vi "SetTIA.vi"(8 "error in (no error)":errorcluster, 11 "Laser Diode Controller in":refnum<class "KLD101.lvclass">) -> (0 "error out":errorcluster, 3 "Laser Diode Controller out":refnum<class "KLD101.lvclass">)   [LabVIEW 2016, in "Laser Diode Controller.lvlib" / "KLD101.lvclass"]
uses:
  KLD101.lvclass
  KLD101.lvclass/KLD101.ctl
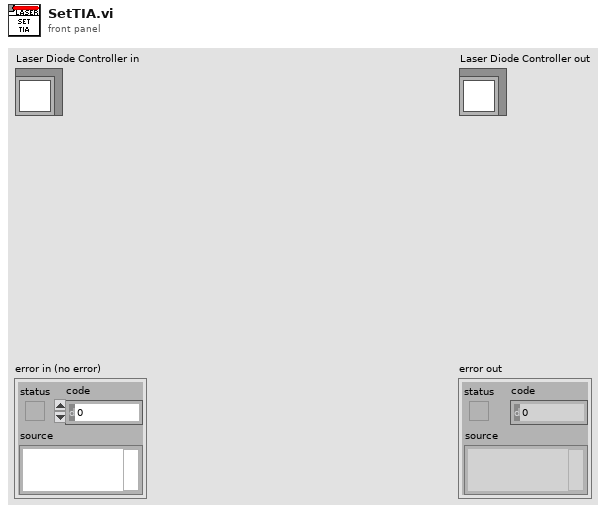
[diagram p1: front panel]
types:
  T1 = typedef "Configuration.lvlib/Config Data.lvclass/LaserMode.ctl" = enum16{"Constant Power", "Constant Current"}
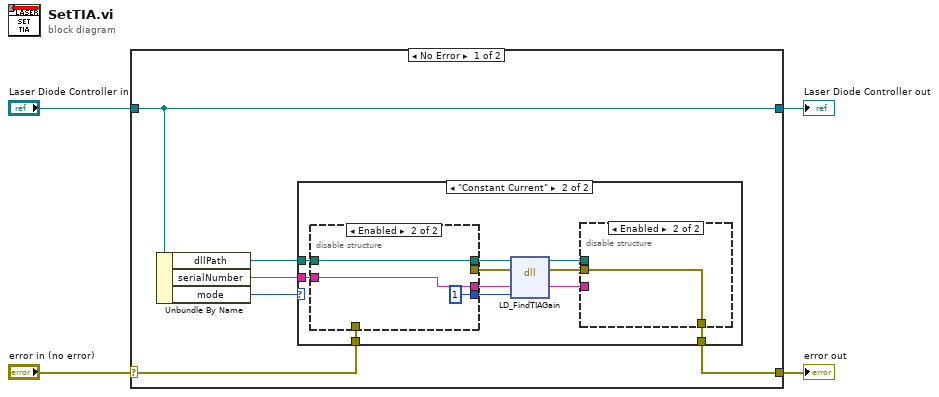
[diagram p0: block diagram]
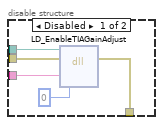
[diagram p3: hidden frame]
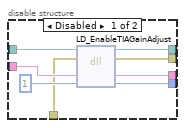
[diagram p4: hidden frame]
diagram:
  n1 = case shown="No Error" "error in (no error)" {
    selector: "error in (no error)" -> [w7 w41]
    tunnel: [w6 w41] -> w3
    tunnel: [w10 w40] -> w1
    tunnel: "Laser Diode Controller in" -> [w10 w40]
    frame No Error {
      n2 = Unbundle By Name(w10) -> ("dllPath"=w9:path, "serialNumber"=w8:string, "mode"=w5:T1)
      n3 = case shown="\"Constant Current\"" w5 {
        tunnel: w9 -> [_ w22]
        tunnel: w8 -> [_ w21]
        tunnel: w7 -> [w11 w13]
        tunnel: [w11 w12] -> w6
        frame "Constant Power", Default {
        }
        frame "Constant Current" {
          n4 = disable-structure shown="Enabled" {
            disable-tunnel: w22 -> [w36 w38]
            disable-tunnel: w21 -> [w34 w39]
            disable-tunnel: [w33 u8 1 ("enableAdjust")] -> w20
            disable-tunnel: [w32 w39] -> w19
            disable-tunnel: [w31 _] -> w18
            disable-tunnel: [w30 w38] -> w17
            disable-tunnel: w13 -> [w29 _]
            frame Disabled {
              n5 = dll-call lib="C:/IDEXX Software/Collimation/data/Thorlabs.MotionControl.KCube.LaserDiode.dll" fn="LD_EnableTIAGainAdjust"(path in=w36, error in=w29, "serialNumber"=w34, "enableAdjust"=u8 1) -> (path out=w30:path, error out=w31:errorcluster, "serialNumber"=w32:string, "enableAdjust"=w33:u8)  [unwired: 2 in]
            }
            frame Enabled {
            }
          }
          n6 = dll-call lib="C:/IDEXX Software/Collimation/data/Thorlabs.MotionControl.KCube.LaserDiode.dll" fn="LD_FindTIAGain"(path in=w17, error in=w18, "serialNumber"=w19, "enable"=w20) -> (path out=w16:path, error out=w15:errorcluster, "serialNumber"=w14:string)  [unwired: 3 in]
          n7 = disable-structure shown="Enabled" {
            disable-tunnel: w16 -> [w27 _]
            disable-tunnel: w15 -> [w26 w28]
            disable-tunnel: w14 -> [w25 _]
            disable-tunnel: [w24 w28] -> w12
            frame Disabled {
              n8 = dll-call lib="C:/IDEXX Software/Collimation/data/Thorlabs.MotionControl.KCube.LaserDiode.dll" fn="LD_EnableTIAGainAdjust"(path in=w27, error in=w26, "serialNumber"=w25, "enableAdjust"=u8 0) -> (error out=w24:errorcluster)  [unwired: 4 in, 1 out]
            }
            frame Enabled {
            }
          }
        }
      }
    }
    frame Error {
    }
  }
  "error out" <- w3
  "Laser Diode Controller out" <- w1
